vi "LVClass_ComputePhaseSet SetZonalPrefs.vi"(0 "ComputePhaseSet in":refnum<class "ComputePhaseSet.lvclass">, 5 "WavefrontSetup.ZonalSetup":T1={"Number of weak iterations"=6, "Number of max iterations"=100, "Residual limit"=5e-05}, 11 "error in (no error)":errorcluster) -> (4 "ComputePhaseSet out":refnum<class "ComputePhaseSet.lvclass">, 15 "error out":errorcluster)   [LabVIEW 2020, in "ComputePhaseSet.lvclass"]
doc: "Set preferences for zonal phase reconstruction.\n\n--------------------------------------------------------------------------------\n\n<B>ComputePhaseSetIn </B> : ComputePhaseSet object.\n<B>ComputePhaseSetOut </B> : ComputePhaseSet object.\n<B>nb_weak_iterations </B> : Maximum number of weak iterations. A weak iteration is an iteration for which\n the variation of the residue from previous iteration is below the\n residual_limit multiplied by the number of microlenses of the Haso.\n<B>nb_max_iterations </B> : Maximum number of iterations.\n<B>residual_limit </B> : Residual variation limit.\n<B>ErrorIn </B> : Error\n<B>ErrorOut </B> : Error\n\n--------------------------------------------------------------------------------"
uses:
  ComputePhaseSet.lvclass
  ZonalPrefs.ctl
  ComputePhaseSet.lvclass/ComputePhaseSet.ctl
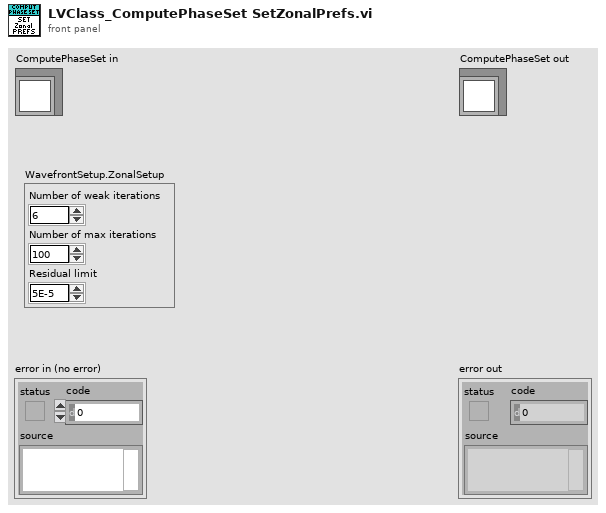
[diagram p1: front panel]
types:
  T1 = typedef "ZonalPrefs.ctl" = cluster{"Number of weak iterations":u16, "Number of max iterations":u32, "Residual limit":sgl}
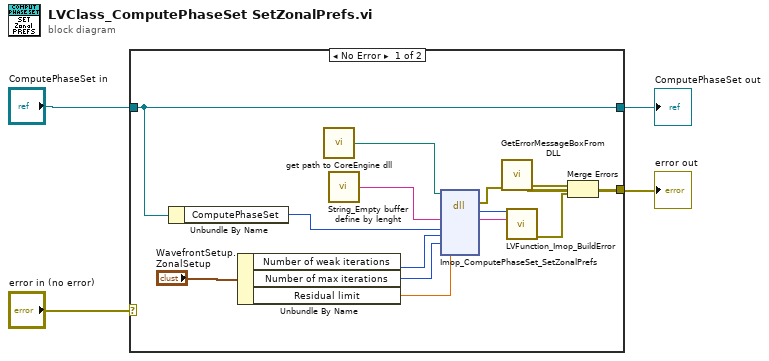
[diagram p0: block diagram]
diagram:
  n1 = case shown="No Error" "error in (no error)" {
    selector: "error in (no error)" -> [_ w20]
    tunnel: [w5 w20] -> w1
    tunnel: [w12 w19] -> w3
    tunnel: "ComputePhaseSet in" -> [w12 w19]
    frame No Error {
      n2 = Unbundle By Name(w12) -> ("ComputePhaseSet"=w11:i32)
      n3 = Unbundle By Name("WavefrontSetup.ZonalSetup") -> ("Number of weak iterations"=w10:u16, "Number of max iterations"=w9:u32, "Residual limit"=w8:sgl)
      n4 = call "get path to CoreEngine dll.vi"() -> ("path to c_interface_vc100.dll"=w15:path)  [unwired: 12 in, 3 out]
      n5 = call "String_Empty buffer define by lenght.vi"() -> ("Empty buffer"=w16:string)  [unwired: 1 in]
      n6 = dll-call lib="D:/2_trunk/Soft_haso/ImOpCoreEngine4_LV2011/DLLs/ImopEngine4_vc100.dll" fn="Imop_ComputePhaseSet_SetZonalPrefs"(path in=w15, "message"=w16, "objet"=w11, "nb_weak_iterations"=w10, "nb_max_iterations"=w9, "residual_limit"=w8) -> (error out=w14:errorcluster, "return type"=w18:i32, "message"=w17:string)  [unwired: 6 in, 1 out]
      n7 = call "GetErrorMessageBoxFromDLL.vi"("error IN"=w14) -> ("error OUT"=w7:errorcluster)  [unwired: 10 in]
      n8 = call "LVFunction_Imop_BuildError.vi"("code"=w18, "String to Prepend to source (\"\")"=w17) -> ("error out"=w6:errorcluster)  [unwired: 13 in]
      n9 = Merge Errors(w7, w6) -> (w5:errorcluster)
    }
    frame Error {
    }
  }
  "error out" <- w1
  "ComputePhaseSet out" <- w3
